vi "Delta init.vi"(5 "robot mode":enum16{"Read", "Write"}(ring), 7 "mode":enum16{"Read", "Write"}(ring), 8 "error in (no error)":errorcluster, 9 "調機參數":T1={"等比調整到角度正確"={"S1"=0.67, "S2"=0.67, "S3"=0.67, "S4"=5.73, "S5"=0.68}, "補償角度到0度是水平"={"S1"=-28.0, "S2"=-25.0, "S3"=-73.0, "S4"=660.0, "S5"=0.0}}, 10 "robot":cluster{"re":dbl, "e":dbl, "rf":dbl, "f":dbl}={"re"=224.0, "e"=60.0, "rf"=145.0, "f"=60.0} {"f" format="%#_13g"; "rf" format="%#_13g"; "e" format="%#_13g"; "re" format="%#_13g"}) -> (0 "error out":errorcluster, 1 "調機參數read":T1, 2 "機構參數read":cluster{"re":dbl, "e":dbl, "rf":dbl, "f":dbl})   [LabVIEW 2019]
uses:
  math/Global 1.vi
  KNRm_ReMi_OS6_436Motor.lvlibp
panel:
  out "視覺參數read":T2
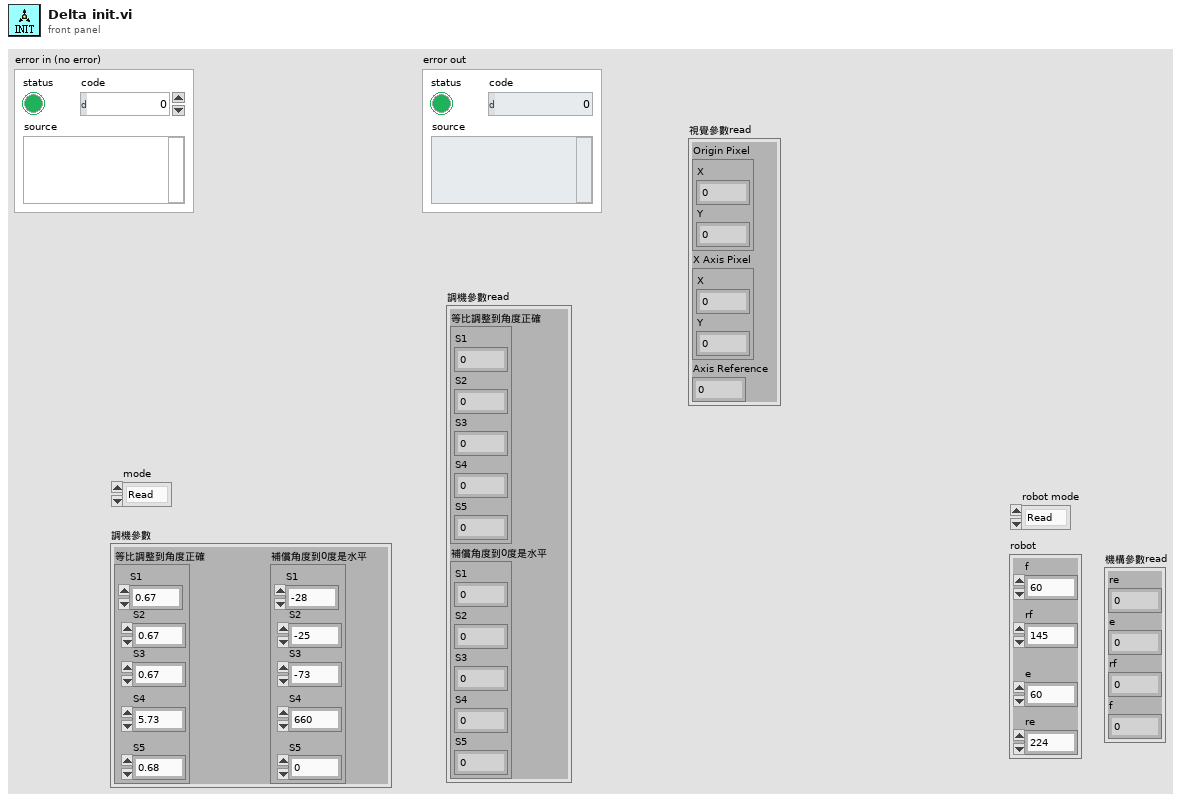
[diagram p1: front panel]
types:
  T1 = cluster{"等比調整到角度正確":cluster{"S1":dbl, "S2":dbl, "S3":dbl, "S4":dbl, "S5":dbl}, "補償角度到0度是水平":cluster{"S1":dbl, "S2":dbl, "S3":dbl, "S4":dbl, "S5":dbl}}
  T2 = cluster{"Origin Pixel":cluster{"X":sgl, "Y":sgl}, "X Axis Pixel":cluster{"X":sgl, "Y":sgl}, "Axis Reference":u32}
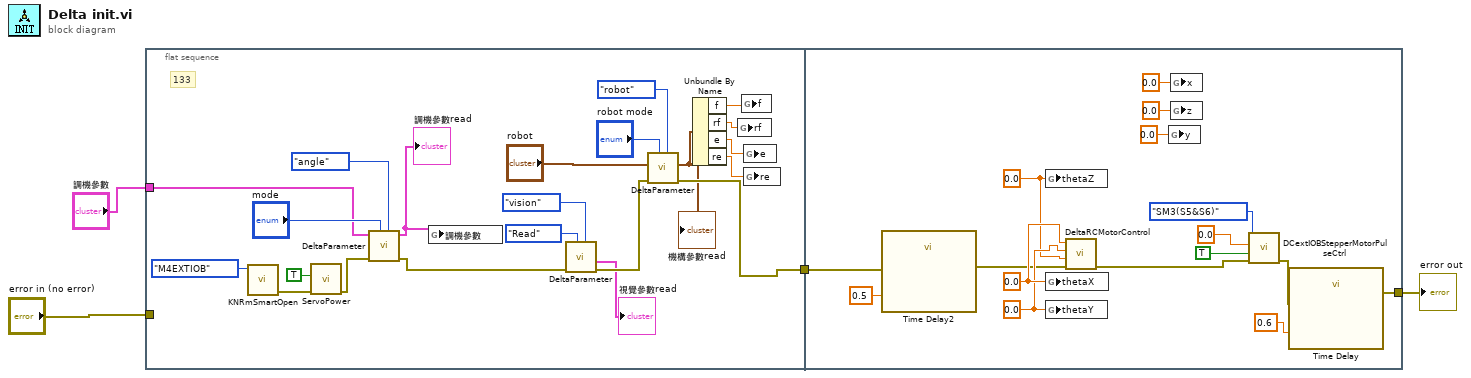
[diagram p0: block diagram]
diagram:
  n1 = flat-sequence {
    tunnel: "error in (no error)" -> [_]
    tunnel: [w23] -> w4
    tunnel: "調機參數" -> [w20]
    tunnel: [w42] -> w2
    tunnel: w4 -> [w33]
    frame #0 {
      # "133"
      n2 = call "KNRmSmartOpen.vi"("INI FPGA MODE"=enum16{"Original", "M4EXTIOB"}."M4EXTIOB") -> ("error out"=w24:errorcluster)  [unwired: 7 in, 3 out]
      n3 = call "ServoPower.vi"("error in (no error)"=w24, "ServoENA"=TRUE) -> ("error out"=w17:errorcluster)  [unwired: 9 in]
      n4 = call "DeltaParameter.vi"("parameter"=enum16{"angle", "robot", "vision"}."angle", "mode"="mode", "error in (no error)"=w17, "調機參數write"=w20) -> ("error out"=w9:errorcluster, "調機參數read"=w22:T1)  [unwired: 3 in, 3 out]
      "調機參數read" <- w22
      n5 = global write "Global 1.vi" "調機參數"(w22) -> ()
      n6 = call "DeltaParameter.vi"("parameter"=enum16{"angle", "robot", "vision"}."vision", "mode"=enum16{"Read", "Write"}."Read", "error in (no error)"=w9) -> ("error out"=w8:errorcluster, "視覺參數read"=→"視覺參數read":T2)  [unwired: 4 in, 3 out]
      n7 = call "DeltaParameter.vi"("parameter"=enum16{"angle", "robot", "vision"}."robot", "mode"="robot mode", "error in (no error)"=w8, "機構參數write"="robot") -> ("error out"=w23:errorcluster, "機構參數read"=w14:cluster{"re":dbl, "e":dbl, "rf":dbl, "f":dbl})  [unwired: 3 in, 3 out]
      "機構參數read" <- w14
      n8 = Unbundle By Name(w14) -> ("f"=w13:dbl, "rf"=w12:dbl, "e"=w11:dbl, "re"=w10:dbl)
      n9 = global write "Global 1.vi" "rf"(w12) -> ()
      n10 = global write "Global 1.vi" "f"(w13) -> ()
      n11 = global write "Global 1.vi" "e"(w11) -> ()
      n12 = global write "Global 1.vi" "re"(w10) -> ()
    }
    frame #1 {
      w29 = 0.0 ("Theta3")
      w30 = 0.0 ("Theta2")
      w31 = 0.0 ("Theta1")
      n13 = call "Time Delay2"("error in (no error)"=w33, "Delay Time (s)"=0.5) -> ("error out"=w28:errorcluster)  [unwired: 9 in]
      n14 = global write "Global 1.vi" "thetaZ"(w29) -> ()
      n15 = global write "Global 1.vi" "thetaX"(w31) -> ()
      n16 = global write "Global 1.vi" "thetaY"(w30) -> ()
      n17 = call "DeltaRCMotorControl.vi"("error in (no error)"=w28, "Theta3"=w29, "Theta2"=w30, "Theta1"=w31) -> ("error out"=w27:errorcluster)  [unwired: 7 in]
      n18 = global write "Global 1.vi" "y"(0.0 ("y")) -> ()
      n19 = global write "Global 1.vi" "x"(0.0 ("x")) -> ()
      n20 = global write "Global 1.vi" "z"(0.0 ("z")) -> ()
      n21 = call "DCextIOBStepperMotorPulseCtrl.vi"("error in"=w27, "ResetCounter"=TRUE, "PulseRate&Dir P/S"=0.0, "Port"=enum16{"SM1(S1&S2)", "SM2(S3&S4)", "SM3(S5&S6)"}."SM3(S5&S6)") -> ("error out"=w37:errorcluster)  [unwired: 6 in, 1 out]
      n22 = call "Time Delay"("error in (no error)"=w37, "Delay Time (s)"=0.6) -> ("error out"=w42:errorcluster)  [unwired: 9 in]
    }
  }
  "error out" <- w2
